vi "CRYGet Auto Delay Curve array.vi"(8 "Polarity":bool, 9 "Additive Info":T4, 10 "Distance Unit":u16) -> (1 "Value Display Array":T3(array[cluster]), 2 "Value Unit Info Out":T2(array[cluster]), 3 "Curve Info Array Out":T1)   [LabVIEW 2013]
uses:
  Typedef Control/CRYAnalysis CurveName Cluster.ctl
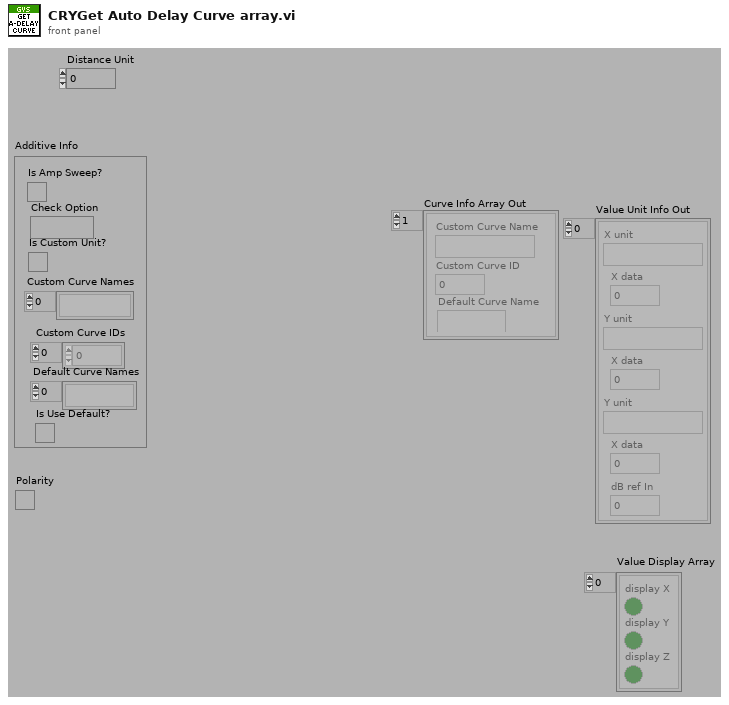
[diagram p1: front panel]
types:
  T1 = typedef "CRYAnalysis CurveName Cluster.ctl" = cluster{"Custom Curve Name":string, "Custom Curve ID":i32, "Default Curve Name":string}[]
  T2 = cluster{"X unit":string, "X data":u16, "Y unit":string, "X data":u16, "Y unit":string, "X data":u16, "dB ref In":dbl}[]
  T3 = cluster{"display X":bool, "display Y":bool, "display Z":bool}[]
  T4 = cluster{"Is Amp Sweep?":bool, "Check Option":string, "Is Custom Unit?":bool, "Custom Curve Names":string[], "Custom Curve IDs":i32[], "Default Curve Names":string[], "Is Use Default?":bool}
  T5 = cluster{"display X":bool, "display Y":bool, "display Z":bool}
  T6 = enum32{"English", "Chinese", "Korean", "Japanese", "Russian", "Chinese traditional"}
  T7 = cluster{"X unit":string, "X data":u16, "Y unit":string, "X data":u16, "Y unit":string, "X data":u16, "dB ref In":dbl}
  T8 = cluster{"X unit":string, "X data":u16, "X unit":string, "X data":u16, "X unit":string, "X data":u16, "dB ref In":dbl}
  T9 = cluster{"X unit":string, "X data":u16, "X unit":string, "X data":u16, "X unit":string, "X data":u16, "dB ref In":dbl}[]
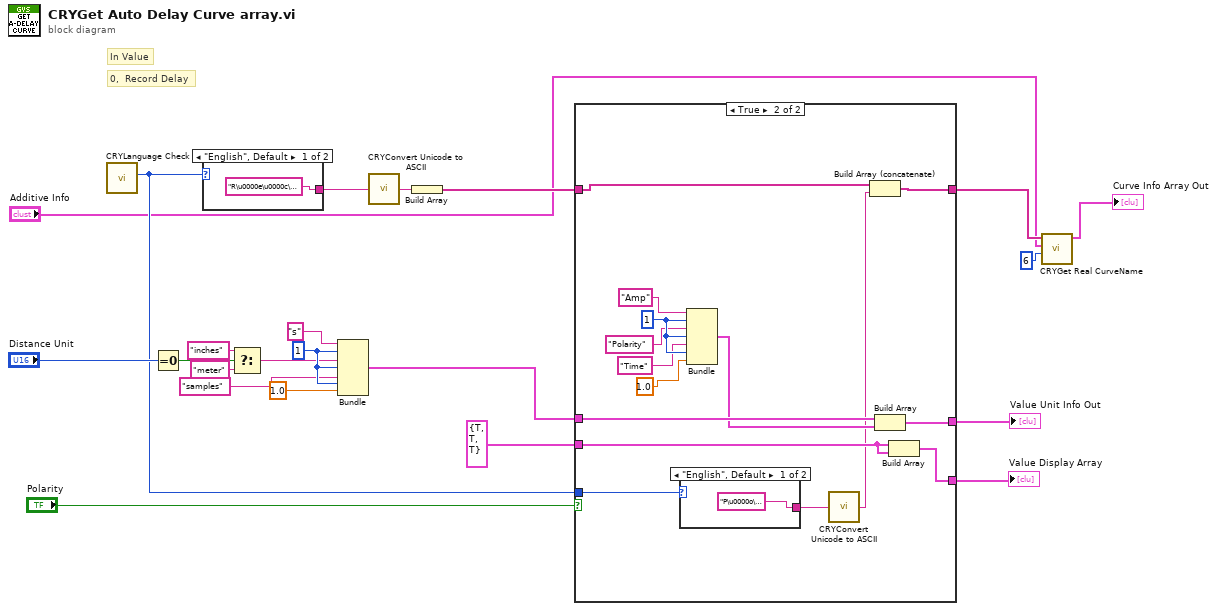
[diagram p0: block diagram]
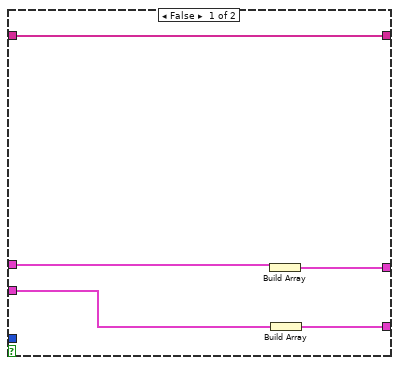
[diagram p2: hidden frame]
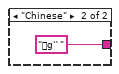
[diagram p3: hidden frame]
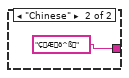
[diagram p4: hidden frame]
diagram:
  w21 = u16 1 ("X data")
  # "In Value"
  # "0,  Record Delay"
  n1 = call "CRYLanguage Check.vi"() -> ("Language"=w10:T6)  [unwired: 10 in, 1 out]
  n2 = Equal To 0?(x="Distance Unit") -> (x = 0?=w15:bool)
  n3 = case shown="\"English\", Default" w10 {
    tunnel: ["R\u0000e\u0000c\u0000o\u0000r\u0000d\u0000 \u0000D\u0000e\u0000l\u0000a\u0000y\u0000" ("message") "ÇÆö^ß" ("message")] -> w13
    frame "English", Default {
    }
    frame "Chinese" {
    }
  }
  n4 = Select(t="inches" ("Y unit"), s=w15, f="meter" ("Y unit")) -> (s? t:f=w16:string)
  n5 = Bundle("X unit"="s", "X data"=w21, "Y unit"=w16, "X data"=w21, "Y unit"="samples", "X data"=w21, "dB ref In"=1.0) -> (w7:T7)  [unwired: 1 in]
  n6 = call "CRYConvert Unicode to ASCII.vi"("Unicode"=w13) -> ("ASCII"=w12:string)  [unwired: 4 in]
  n7 = Build Array(w12) -> (w5:string[])
  n8 = case shown="True" "Polarity" {
    tunnel: w10 -> [_ w43]
    tunnel: T5 {"display X"=TRUE, "display Y"=TRUE, "display Z"=TRUE} -> [w29 w42]
    tunnel: [w28 w41] -> w8
    tunnel: w7 -> [w27 w40]
    tunnel: [w26 w39] -> w6
    tunnel: w5 -> [w25 w32]
    tunnel: [w25 w30] -> w3
    frame False {
      n9 = Build Array(w27) -> (w26:T2)
      n10 = Build Array(w29) -> (w28:T3)
    }
    frame True {
      w38 = u16 1 ("X data")
      n11 = case shown="\"English\", Default" w43 {
        tunnel: ["P\u0000o\u0000l\u0000a\u0000r\u0000i\u0000t\u0000y\u0000" ("message") "g'`" ("message")] -> w44
        frame "English", Default {
        }
        frame "Chinese" {
        }
      }
      n12 = Bundle("X unit"="Amp", "X data"=w38, "X unit"="Polarity", "X data"=w38, "X unit"="Time", "X data"=w38, "dB ref In"=1.0) -> (w36:T8)  [unwired: 1 in]
      n13 = call "CRYConvert Unicode to ASCII.vi"("Unicode"=w44) -> ("ASCII"=w31:string)  [unwired: 4 in]
      n14 = Build Array (concatenate)(w32, w31) -> (w30:string[])
      n15 = Build Array(w40, w36) -> (w39:T9)
      n16 = Build Array(w42, w42) -> (w41:T3)
    }
  }
  "Value Display Array" <- w8
  "Value Unit Info Out" <- w6
  n17 = call "CRYGet Real CurveName.vi"("Key No"=6, "Additive Info"="Additive Info", "CurveArrayByType"=w3) -> ("Curve Info Array Out"=→"Curve Info Array Out":T1)  [unwired: 8 in]
